vi "FindDecoPosition.vi"(1 "Text":string, 2 "Decos[]":refnum<vi>[](array[refnum])) -> (0 "Position":T1)   [LabVIEW 2018]
doc: "返回与制定的文本内容匹配的装饰文本控件的位置"
uses:
  <vilib>/Utility/miscctls.llb/LVPositionTypeDef.ctl
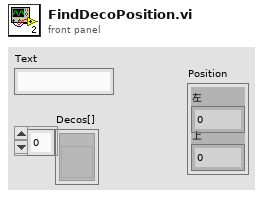
[diagram p1: front panel]
types:
  T1 = typedef "LVPositionTypeDef.ctl" = cluster{"Left":i32, "Top":i32}
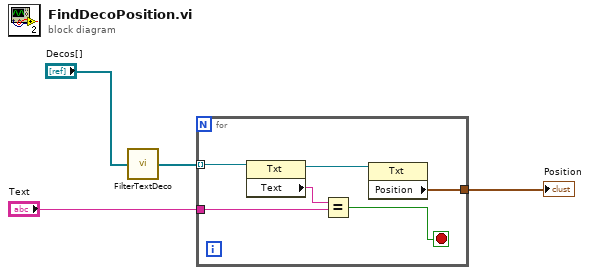
[diagram p0: block diagram]
diagram:
  n1 = call "FilterTextDeco.vi"("Decos[]"="Decos[]") -> ("TextDecos"=w3:refnum<vi>[])
  n2 = for {
    tunnel: w3 -> [w10] mode=indexing
    tunnel: [w6] -> w1
    tunnel: "Text" -> [w5]
    stop <- w7 stop-if-true
    n3 = property class="Txt"(reference=w10) -> (reference out=w8:refnum<vi>, "Text"=w9:string)  [unwired: 1 in, 1 out]
    n4 = Equal?(x=w9, y=w5) -> (x = y?=w7:bool)
    n5 = property class="Txt"(reference=w8) -> ("Position"=w6:T1)  [unwired: 1 in, 2 out]
  }
  "Position" <- w1
